vi "Host-UART-State-Machine-Tester.vi"() -> ()   [LabVIEW 2017]
uses:
  UART.States.ctl
  <vilib>/FPGAPlugInAG/Dynamic/niLvFpga_Download_Dynamic.vi
  <vilib>/Utility/error.llb/Error Cluster From Error Code.vi
  <vilib>/rvi/errors/niLvFpgaAdjustHostInterfaceError.vi
  <vilib>/FPGAPlugInAG/Dynamic/niLvFpga_Run_Dynamic.vi
  <vilib>/FPGAPlugInAG/Dynamic/niLvFpga_Close_Dynamic.vi
  <vilib>/rvi/interface/nirviMethod/nirviMethod.xnode
  <vilib>/rvi/interface/nirviReadWriteControl/nirviReadWriteControl.xnode
  <vilib>/rvi/interface/nirviCloseFPGA/nirviCloseFPGA.xnode
  <vilib>/FPGAPlugInAG/Dynamic/niLvFpga_ReadFifo_Dynamic.vi
  <vilib>/rvi/errors/niLvFpgaMergeErrorWithErrorCode.vi
  NiFpgaLv.dll
  <vilib>/rvi/interface/Simulation/niFpgaSimulationCallBeginRW.vi
  <vilib>/FPGAPlugInAG/Dynamic/niLvFpga_WriteFifo_Dynamic.vi
panel:
  out "FPGA\nReady":bool
  in  "Download\nBitfile?":bool=TRUE
  in  "Data to Send":string="A"
  in  "Receive":bool
  in  "Transmit":bool
  in  "Bitfile path":path
  out "Data Received":string
  out "error out":errorcluster
  in  "stop":bool
  in  "error in":errorcluster
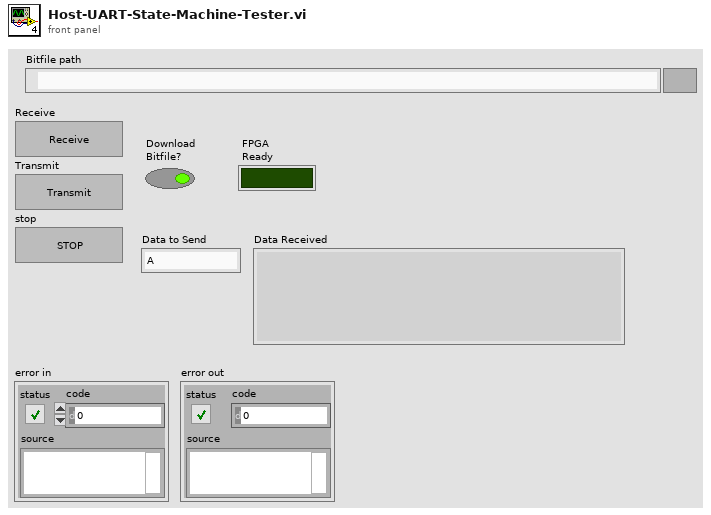
[diagram p1: front panel]
types:
  T1 = typedef "UART.States.ctl" = enum16{"Open-Fpga", "Poll-RX", "Transmit", "Close-Fpga"}
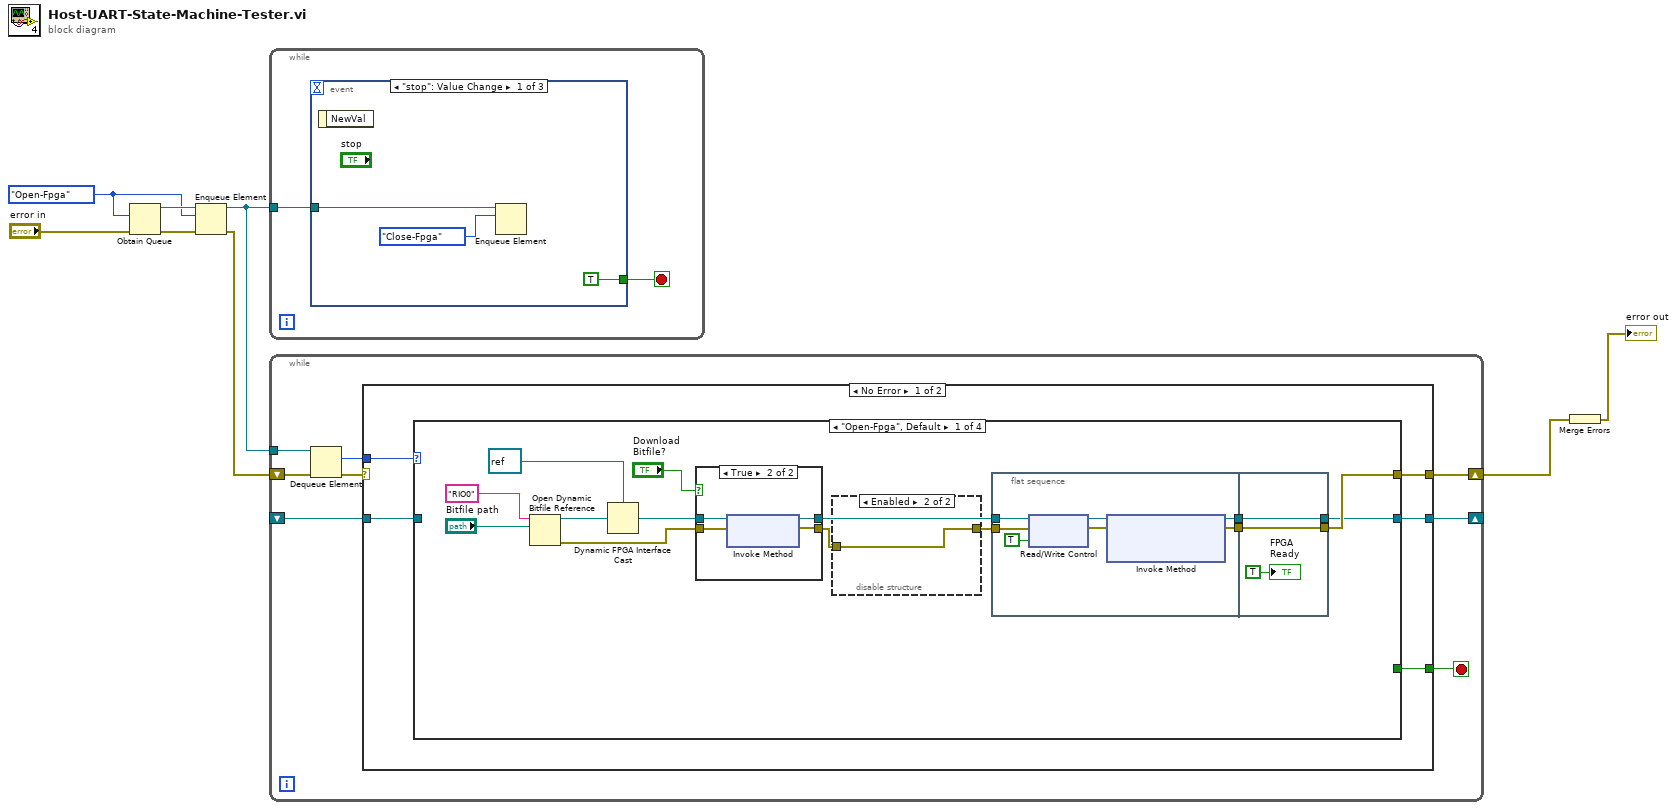
[diagram p0: block diagram]
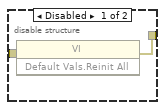
[diagram p2: hidden frame]
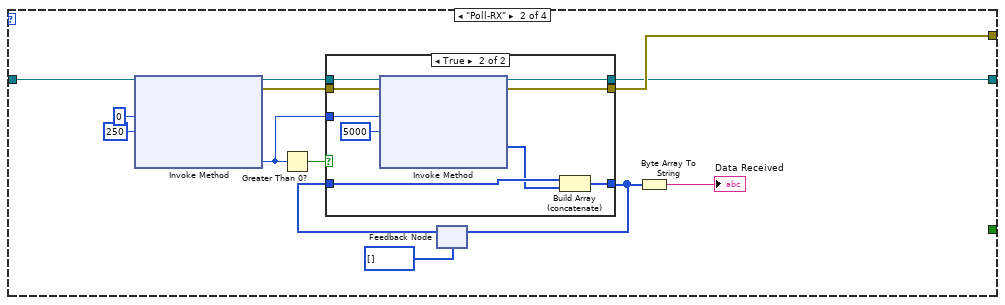
[diagram p4: hidden frame]
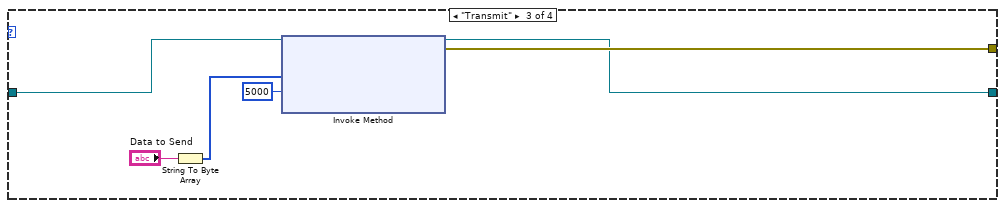
[diagram p6: hidden frame]
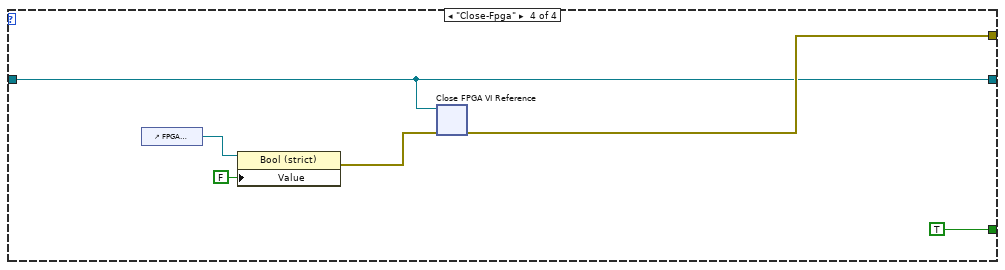
[diagram p7: hidden frame]
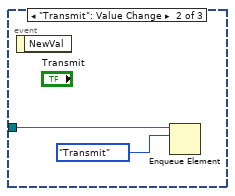
[diagram p9: hidden frame]
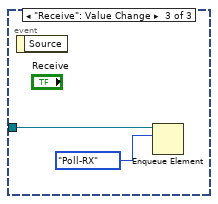
[diagram p10: hidden frame]
diagram:
  w5 = UART.States."Open-Fpga"
  n1 = Obtain Queue(element data type=w5, error in (no error)="error in") -> (queue out=w7:refnum<queue>, error out=w6:errorcluster)  [unwired: 3 in, 1 out]
  n2 = Enqueue Element(queue=w7, element=w5, error in (no error)=w6) -> (queue out=w4:refnum<queue>, error out=w3:errorcluster)  [unwired: 1 in, 1 out]
  n3 = while {
    tunnel: w4 -> [w10]
    stop <- w9 stop-if-true
    n4 = event shown="[0] \"stop\": Value Change" {
      selector: _ -> [_ _ _]
      dyn-events: _ -> [_ _ _]
      timeout: _ -> [_ _ _]
      tunnel: w10 -> [w13 w14 w16]
      tunnel: [TRUE _ _] -> w9
      event "stop": Value Change {
        n5 = event-data() -> ()  [unwired: 1 in, 1 out]
        n6 = Enqueue Element(queue=w13, element=UART.States."Close-Fpga") -> ()  [unwired: 2 in, 3 out]
      }
      event "Transmit": Value Change {
        n7 = event-data() -> ()  [unwired: 1 in, 1 out]
        n8 = Enqueue Element(queue=w14, element=UART.States."Transmit") -> ()  [unwired: 2 in, 3 out]
      }
      event "Receive": Value Change {
        n9 = event-data() -> ()  [unwired: 1 in, 1 out]
        n10 = Enqueue Element(queue=w16, element=UART.States."Poll-RX") -> ()  [unwired: 2 in, 3 out]
      }
    }
  }
  n11 = while {
    tunnel: w4 -> [w23]
    shift-right: [w20] -> w2
    shift-left: w3 -> [w22]
    shift-right: [w19] -> _
    shift-left: _ -> [w18]
    stop <- w21 stop-if-true
    n12 = Dequeue Element(queue=w23, error in (no error)=w22) -> (element=w24:T1, error out=w25:errorcluster)  [unwired: 1 in, 2 out]
    n13 = case shown="No Error" w25 {
      selector: w25 -> [_ w102]
      tunnel: w24 -> [w30 _]
      tunnel: [w29 _] -> w21
      tunnel: [w28 w102] -> w20
      tunnel: w18 -> [w27 w101]
      tunnel: [w26 w101] -> w19
      frame No Error {
        n14 = case shown="\"Open-Fpga\", Default" w30 {
          tunnel: [_ _ _ TRUE] -> w29
          tunnel: [w44 w70 w93 w99] -> w28
          tunnel: w27 -> [_ w64 w89 w98]
          tunnel: [w42 w65 w90 w98] -> w26
          frame "Open-Fpga", Default {
            n15 = Open Dynamic Bitfile Reference(0:"RIO0" ("Device address"), 1:"Bitfile path") -> (5:w35:refnum<k20>, 8:w33:errorcluster)  [unwired: 3 in]
            n16 = Dynamic FPGA Interface Cast(Session In=refnum<k20> refnum ("FPGA Interface"), Type=w35) -> (Session Out=w34:refnum<k20>)
            n17 = case shown="True" "Download\nBitfile?" {
              tunnel: w34 -> [w58 w63]
              tunnel: [w58 w62] -> w43
              tunnel: w33 -> [w59 w61]
              tunnel: [w59 w60] -> w38
              frame False {
              }
              frame True {
                n18 = xnode "Invoke Method"("FPGA VI Reference In"=w63, "error in"=w61) -> ("FPGA VI Reference Out"=w62:refnum<k20>, "error out"=w60:errorcluster)
              }
            }
            n19 = disable-structure shown="Enabled" {
              disable-tunnel: w38 -> [w46 w47]
              disable-tunnel: [w45 w47] -> w37
              frame Disabled {
                n20 = invoke class="VI" method="Default Vals.Reinit All"(error in=w46) -> (error out=w45:errorcluster)  [unwired: 2 in, 2 out]
              }
              frame Enabled {
              }
            }
            n21 = flat-sequence {
              tunnel: [w51] -> w40
              tunnel: [w49] -> w39
              tunnel: w43 -> [w50]
              tunnel: w37 -> [w48]
              tunnel: [w56] -> w42
              tunnel: [w57] -> w44
              tunnel: w40 -> [w57]
              tunnel: w39 -> [w56]
              frame #0 {
                n22 = xnode "Read/Write Control"("FPGA VI Reference In"=w50, "error in"=w48, "reset_rtl"=TRUE) -> ("FPGA VI Reference Out"=w54:refnum<k20>, "error out"=w52:errorcluster)
                n23 = xnode "Invoke Method"("FPGA VI Reference In"=w54, "error in"=w52) -> ("FPGA VI Reference Out"=w49:refnum<k20>, "error out"=w51:errorcluster)  [unwired: 1 in]
              }
              frame #1 {
                "FPGA\nReady" <- TRUE ("FPGA\nReady")
              }
            }
          }
          frame "Poll-RX" {
            n24 = xnode "Invoke Method"("FPGA VI Reference In"=w64, "Number of Elements"=u32 0, "Timeout (ms)"=250) -> ("FPGA VI Reference Out"=w73:refnum<k20>, "error out"=w72:errorcluster, "Elements Remaining"=w71:u32)  [unwired: 1 in, 1 out]
            n25 = Greater Than 0?(x=w71) -> (x > 0?=w74:bool)
            n26 = feedback #1(u8[] []) -> (w69:u8[])
            n27 = case shown="True" w74 {
              tunnel: w73 -> [w77 w88]
              tunnel: w72 -> [w78 w87]
              tunnel: w71 -> [_ w86]
              tunnel: w69 -> [w79 w84]
              tunnel: [w79 w82] -> w67
              tunnel: [w77 w81] -> w65
              tunnel: [w78 w80] -> w70
              frame False {
              }
              frame True {
                n28 = xnode "Invoke Method"("FPGA VI Reference In"=w88, "error in"=w87, "Number of Elements"=w86, "Timeout (ms)"=5000) -> ("FPGA VI Reference Out"=w81:refnum<k20>, "error out"=w80:errorcluster, "Data"=w83:u8[])  [unwired: 1 out]
                n29 = Build Array (concatenate)(w84, w83) -> (w82:u8[])
              }
            }
            n30 = feedback-in #1(w67) -> ()
            n31 = Byte Array To String(unsigned byte array=w67) -> (string=→"Data Received":string)
          }
          frame "Transmit" {
            n32 = String To Byte Array(string="Data to Send") -> (unsigned byte array=w92:u8[])
            n33 = xnode "Invoke Method"("FPGA VI Reference In"=w89, "Data"=w92, "Timeout (ms)"=5000) -> ("FPGA VI Reference Out"=w90:refnum<k20>, "error out"=w93:errorcluster)  [unwired: 1 in, 1 out]
          }
          frame "Close-Fpga" {
            n34 = control-ref of="FPGA\nReady"() -> (w97:refnum<vi>)
            n35 = property class="Bool (strict)"(reference=w97, "Value"=FALSE) -> (error out=w95:errorcluster)  [unwired: 1 in, 1 out]
            n36 = xnode "Close FPGA VI Reference"("FPGA VI Reference In"=w98, "error in"=w95) -> ("error out"=w99:errorcluster)
          }
        }
      }
      frame Error {
      }
    }
  }
  n37 = Merge Errors(w2) -> (→"error out":errorcluster)
